vi "AeroQuadUploader.vi"(11 "Com Port":refnum<visa-resource-name>="<Select Com Port>") -> (3 "Com Port Out":refnum<visa-resource-name>)   [LabVIEW 2010]
uses:
  <vilib>/Utility/config.llb/Config Data RefNum.ctl
  <vilib>/Utility/config.llb/Read Key (Double).vi
  <vilib>/Utility/config.llb/Read Key (Boolean).vi
  <vilib>/Utility/config.llb/Read Key (Path).vi
  <vilib>/Utility/config.llb/Read Key (String).vi
  <vilib>/Utility/config.llb/Write Key (Path).vi
  <vilib>/Utility/config.llb/Write Key (Boolean).vi
  <vilib>/Utility/config.llb/NI_LVConfig.lvlib
panel:
  in  "Settings":bool
  in  "Update":bool
  in  "Done":bool
  in  "Upload":bool
  in  "Flight Control Board":u16(ring) items=["AeroQuad v2.1", "AeroQuad v2.0", "AeroQuad Mini", "AeroQuad v1.8 or greater", "AeroQuad v1.0", "AeroQuad v1.0 with IDG gyro", "Wii sensors", "Paris v3", "AeroQuad v1.0 with Arduino Mega", "AeroQuad with Arduino Mega and Wii sensors", "ArduCopter", "AeroQuad with CHR6DM", "APM/OilPan with CHR6DM"]
  in  "Next":bool
  in  "Previous":bool
  in  "FlightConfig":u16(ring) caption="Flight Configuration" items=["Quad X", "Quad +", "Y4", "Tri", "Hexa X", "Hexa +", "Y6", "Octo X", "Octo +", "Octo X8X"]
  out "Description":string
  in  "Options":i32(listbox) caption="Flight Options"
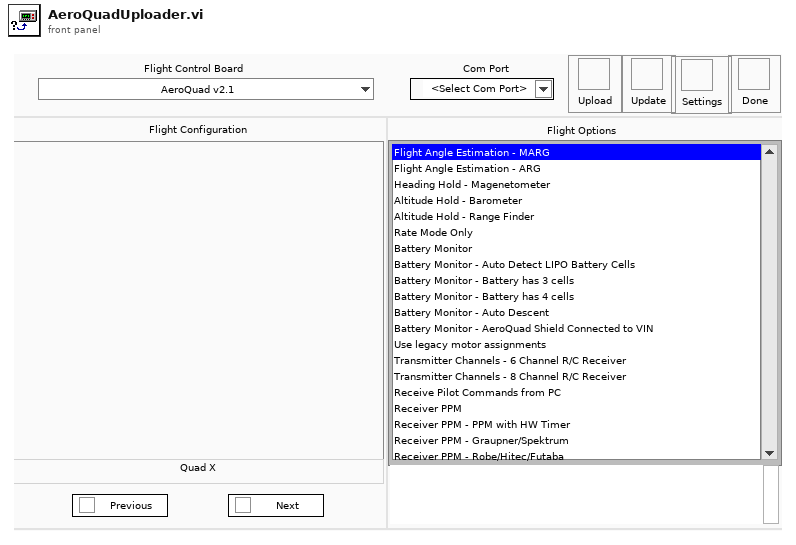
[diagram p1: front panel]
types:
  T1 = typedef "NI_LVConfig.lvlib/Config Data RefNum.ctl" = refnum<k1>
  T2 = cluster{"Error":errorcluster, "ConfigRef":T1, "OptionName":string[], "OptionDesc":string[], "FlightBoard":string[], "ValidOptions":string[][], "ValidBoards":string[], "OptionID":string[], "DefaultOptions":string[][], "DefaultBoards":string[], "FlightSWPath":path, "IDEPath":path, "Debug":bool, "TempPath":path, "Processors":string[][], "ProcessorID":string[], "ConfigID":string[], "ConfigName":string[], "WorkingPath":path, "DebugMsg":bool, "MCU":string, "Mac":bool, "Delay":dbl}
  T3 = enum16{"Left Button", "Center Button", "Right Button", "Window Close"}
  T4 = enum32{"invalid app kind", "Development System", "Run Time System", "Student Edition", "Embedded LabVIEW", "Evaluation", "Custom"}
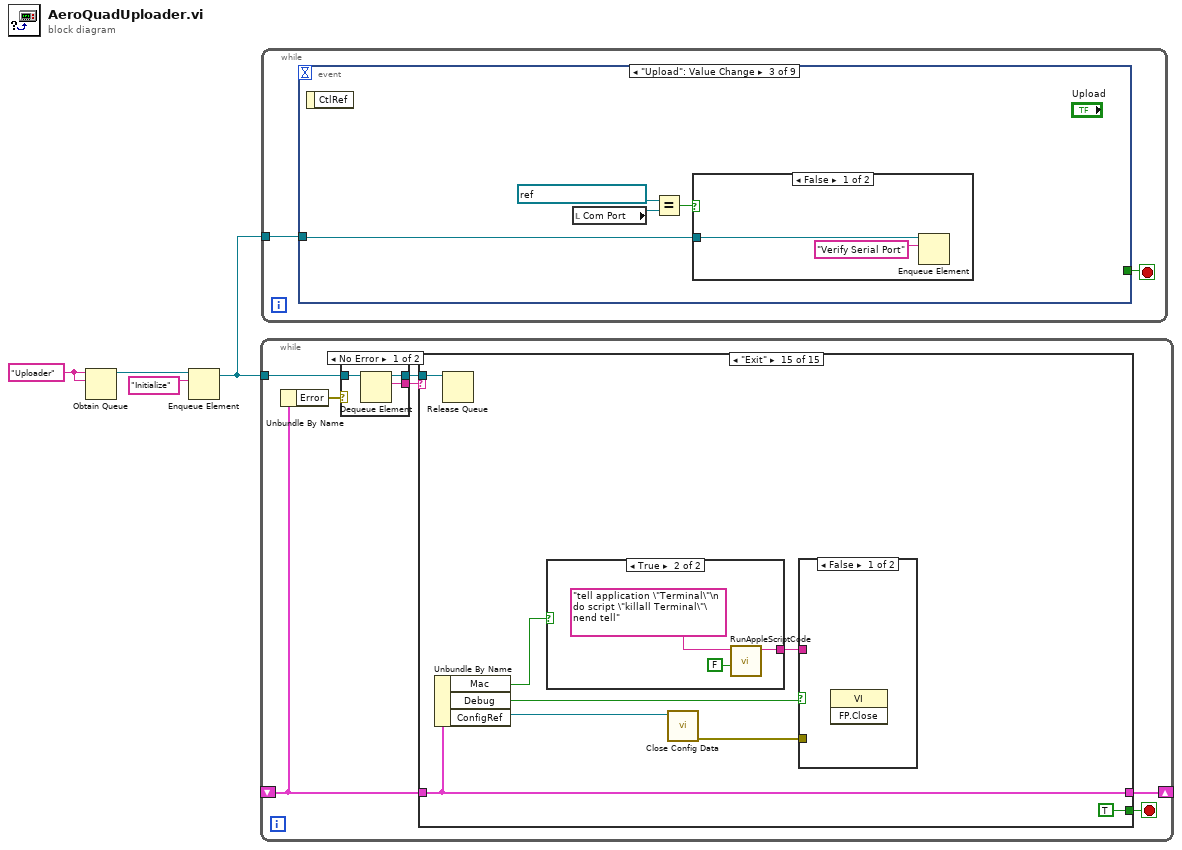
[diagram p0: block diagram]
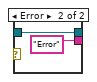
[diagram p2: hidden frame]
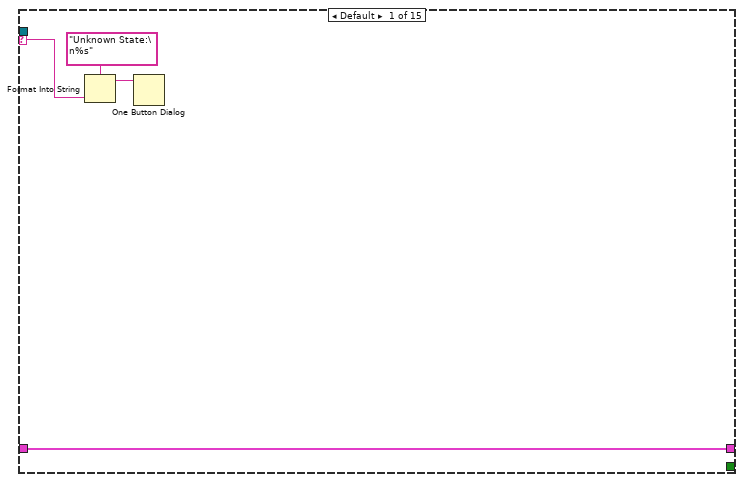
[diagram p3: hidden frame]
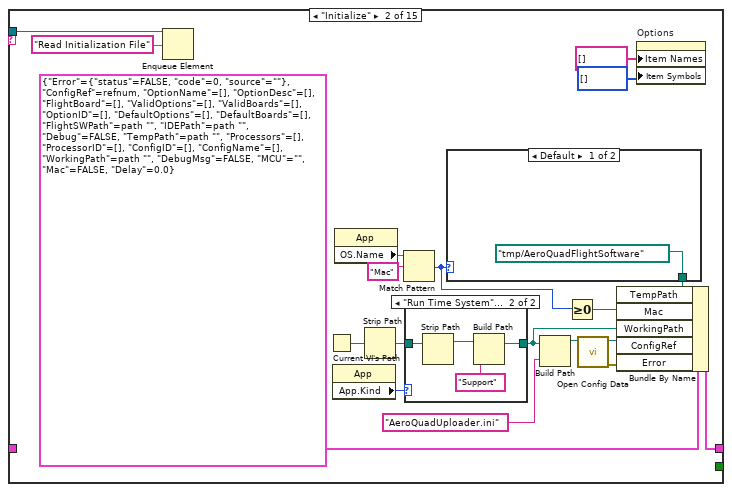
[diagram p4: hidden frame]
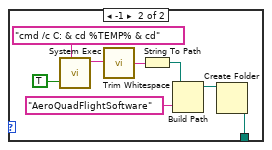
[diagram p5: hidden frame]
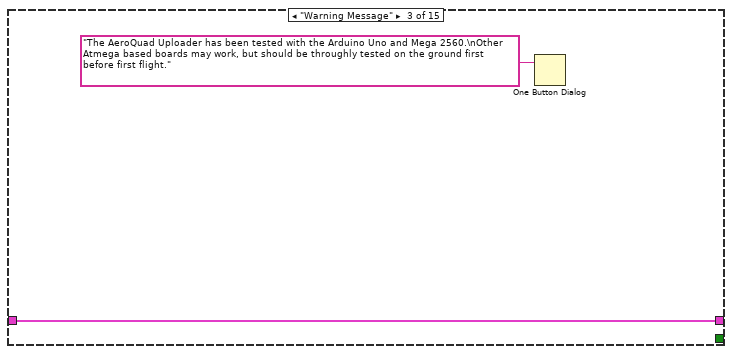
[diagram p7: hidden frame]
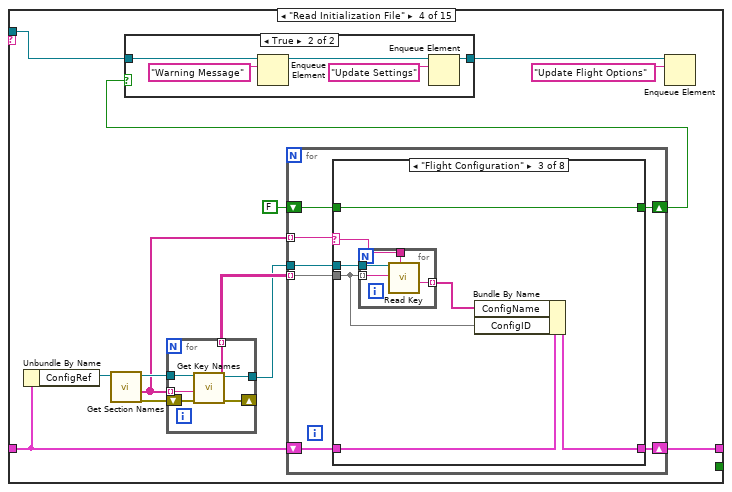
[diagram p8: hidden frame]
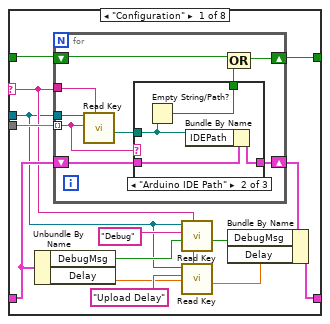
[diagram p10: hidden frame]
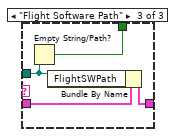
[diagram p12: hidden frame]
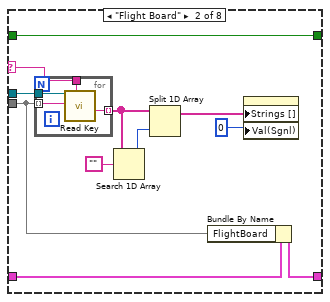
[diagram p13: hidden frame]
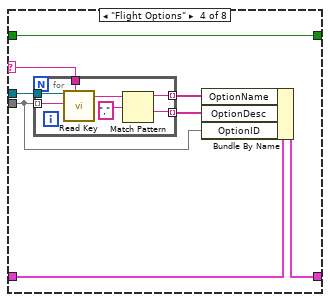
[diagram p14: hidden frame]
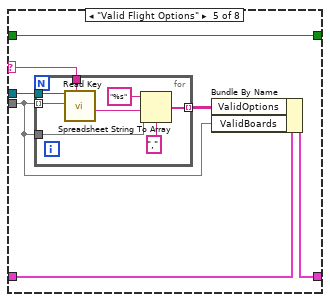
[diagram p15: hidden frame]
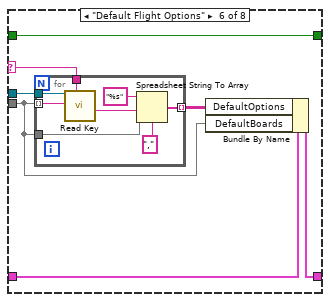
[diagram p16: hidden frame]
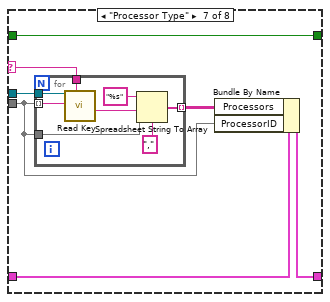
[diagram p17: hidden frame]
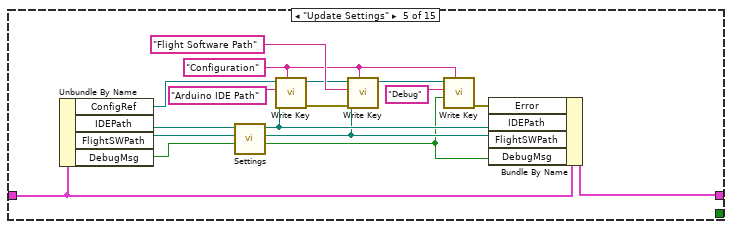
[diagram p19: hidden frame]
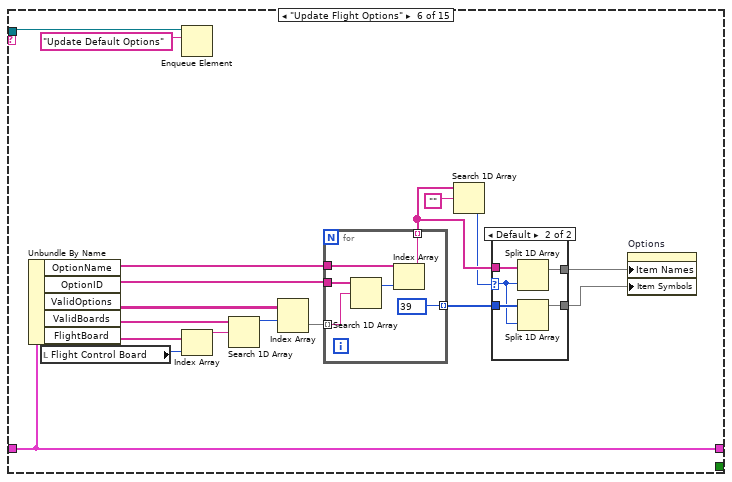
[diagram p20: hidden frame]
diagram:
  w4 = "Uploader" ("name (unnamed)")
  n1 = Obtain Queue(name (unnamed)=w4, element data type=w4) -> (queue out=w3:refnum<queue>)  [unwired: 3 in, 2 out]
  n2 = Enqueue Element(queue=w3, element="Initialize") -> (queue out=w1:refnum<queue>)  [unwired: 2 in, 2 out]
  n3 = while {
    tunnel: w1 -> [w11]
    shift-right: [w8] -> _
    shift-left: _ -> [w7]
    stop <- w9 stop-if-true
    n4 = Unbundle By Name(w7) -> ("Error"=w6:errorcluster)
    n5 = case shown="No Error" w6 {
      tunnel: w11 -> [w14 w15]
      tunnel: [w13 "Error" ("name (unnamed)")] -> w10
      tunnel: [w12 w15] -> w5
      frame No Error {
        n6 = Dequeue Element(queue=w14) -> (queue out=w12:refnum<queue>, element=w13:string)  [unwired: 2 in, 2 out]
      }
      frame Error {
      }
    }
    n7 = case shown="\"Exit\"" w10 {
      tunnel: w5 -> [_ w31 _ w57 _ w226 _ _ w290 w345 w393 w446 _ w586 w597]
      selector: w10 -> [w18 _ _ _ _ _ _ _ _ _ _ _ _ _ _]
      tunnel: [_ _ _ _ _ _ _ _ _ _ _ _ _ _ TRUE] -> w9
      tunnel: [w20 w33 w55 w61 w224 w242 w269 w287 w288 w343 w389 w448 w505 w589 w599] -> w8
      tunnel: w7 -> [w20 _ w55 w62 w223 w242 w269 w287 w288 w340 w390 w449 w506 w590 w599]
      frame Default {
        n8 = Format Into String(format string="Unknown State:\n%s", w18) -> (resulting string=w17:string)  [unwired: 2 in, 1 out]
        n9 = One Button Dialog(message=w17) -> ()  [unwired: 1 in, 1 out]
      }
      frame "Initialize" {
        n10 = Enqueue Element(queue=w31, element="Read Initialization File") -> ()  [unwired: 2 in, 3 out]
        n11 = Current VI's Path() -> (path=w37:path)
        n12 = property class="App"() -> ("App.Kind"=w35:T4)  [unwired: 2 in, 2 out]
        n13 = property class="App"() -> ("OS.Name"=w25:string)  [unwired: 2 in, 2 out]
        n14 = Strip Path(path=w37) -> (stripped path=w36:path)  [unwired: 1 out]
        n15 = Match Pattern(string=w25, regular expression="Mac") -> (offset past match=w22:i32)  [unwired: 1 in, 3 out]
        n16 = case shown="\"Run Time System\", Default" w35 {
          tunnel: w36 -> [w49 w53]
          tunnel: [w49 w52] -> w26
          frame "Development System" {
          }
          frame "Run Time System", Default {
            n17 = Strip Path(path=w53) -> (stripped path=w51:path)  [unwired: 1 out]
            n18 = Build Path(base path=w51, name or relative path="Support") -> (appended path=w52:path)
          }
        }
        n19 = case shown="Default" w22 {
          tunnel: [path "/tmp/AeroQuadFlightSoftware" ("created path") w42] -> w23
          frame Default {
          }
          frame -1 {
            n20 = call <vilib>:"System Exec.vi"("run minimized? (F)"=TRUE, "command line"="cmd /c C: & cd %TEMP% & cd") -> ("standard output"=w44:string)  [unwired: 6 in, 3 out]
            n21 = call <vilib>:"Trim Whitespace.vi"("string"=w44) -> ("trimmed string"=w43:string)  [unwired: 1 in]
            n22 = String To Path(string=w43) -> (path=w46:path)
            n23 = Build Path(base path=w46, name or relative path="AeroQuadFlightSoftware") -> (appended path=w45:path)
            n24 = Create Folder(path (use dialog)=w45) -> (created path=w42:path)  [unwired: 2 in, 2 out]
          }
        }
        n25 = Build Path(base path=w26, name or relative path="AeroQuadUploader.ini") -> (appended path=w39:path)
        n26 = Greater Or Equal To 0?(x=w22) -> (x >= 0?=w21:bool)
        n27 = call <vilib>:"Open Config Data.vi"("configuration file path"=w39) -> ("error out"=w32:errorcluster, "refnum"=w27:T1)  [unwired: 8 in, 1 out]
        n28 = Bundle By Name(cluster=T2 {"Error"={"status"=FALSE, "code"=0, "source"=""}, "ConfigRef"=refnum, "OptionName"=[], "OptionDesc"=[], "FlightBoard"=[], "ValidOptions"=[], "ValidBoards"=[], "OptionID"=[], "DefaultOptions"=[], "DefaultBoards"=[], "FlightSWPath"=path "", "IDEPath"=path "", "Debug"=FALSE, "TempPath"=path "", "Processors"=[], "ProcessorID"=[], "ConfigID"=[], "ConfigName"=[], "WorkingPath"=path "", "DebugMsg"=FALSE, "MCU"="", "Mac"=FALSE, "Delay"=0.0}, "TempPath"=w23, "Mac"=w21, "WorkingPath"=w26, "ConfigRef"=w27, "Error"=w32) -> (w33:T2)
        n29 = property on="Options" class="LstBox (strict)"("Item Names"=string[] [], "Item Symbols"=i32[] []) -> ()  [unwired: 2 in, 2 out]
      }
      frame "Warning Message" {
        n30 = One Button Dialog(message="The AeroQuad Uploader has been tested with the Arduino Uno and Mega 2560.\nOther Atmega based boards may work, but should be throughly tested on the ground first before first flight.") -> ()  [unwired: 1 in, 1 out]
      }
      frame "Read Initialization File" {
        n31 = Unbundle By Name(w62) -> ("ConfigRef"=w64:T1)
        n32 = call <vilib>:"Get Section Names.vi"("refnum"=w64) -> ("error out"=w65:errorcluster, "section names"=w66:string[], "refnum out"=w68:T1)  [unwired: 8 in]
        n33 = for {
          tunnel: w68 -> [w206]
          tunnel: w66 -> [w205] mode=indexing
          shift-right: [w204] -> _
          shift-left: w65 -> [w207]
          tunnel: [w203] -> w63
          tunnel: [w202] -> w67 mode=indexing
          n34 = call <vilib>:"Get Key Names.vi"("section"=w205, "error in (no error)"=w207, "refnum"=w206) -> ("error out"=w204:errorcluster, "key names"=w202:string[], "refnum out"=w203:T1)  [unwired: 5 in, 1 out]
        }
        n35 = for {
          tunnel: w66 -> [w81] mode=indexing
          tunnel: w67 -> [w80] mode=indexing
          tunnel: w63 -> [w79]
          shift-right: [w77] -> w61
          shift-left: w62 -> [w78]
          shift-right: [w75] -> w56
          shift-left: FALSE -> [w76]
          n36 = case shown="\"Flight Configuration\"" w81 {
            selector: w81 -> [w86 w123 w134 w147 w160 w175 w190 _]
            tunnel: w80 -> [w95 w119 w131 w141 w156 w171 w186 _]
            tunnel: w79 -> [w82 w124 w135 w146 w161 w176 w191 _]
            tunnel: w78 -> [w90 w121 w133 w145 w159 w174 w189 w201]
            tunnel: [w92 w120 w132 w144 w158 w173 w188 w201] -> w77
            tunnel: w76 -> [w88 w114 w129 w140 w155 w170 w185 w200]
            tunnel: [w87 w114 w129 w140 w155 w170 w185 w200] -> w75
            frame "Configuration" {
              n37 = Unbundle By Name(w90) -> ("DebugMsg"=w89:bool, "Delay"=w84:dbl)
              n38 = for {
                tunnel: w82 -> [w104]
                tunnel: w86 -> [w103]
                tunnel: w95 -> [w100] mode=indexing
                shift-right: [w101] -> w93
                shift-left: w90 -> [w102]
                shift-right: [w97] -> w87
                shift-left: w88 -> [w98]
                n39 = call-poly <vilib>:"Read Key.vi"("section"=w103, "key"=w100, "refnum"=w104) -> ("value"=w99:path)  [unwired: 5 in, 3 out]
                n40 = case shown="\"Arduino IDE Path\"" w100 {
                  tunnel: w102 -> [w105 w109 w113]
                  tunnel: [w105 w108 w112] -> w101
                  tunnel: w99 -> [_ w107 w111]
                  tunnel: [_ w106 w110] -> w96
                  frame Default {
                  }
                  frame "Arduino IDE Path" {
                    n41 = Empty String/Path?(string/path=w107) -> (empty?=w106:bool)
                    n42 = Bundle By Name(cluster=w109, "IDEPath"=w107) -> (w108:T2)
                  }
                  frame "Flight Software Path" {
                    n43 = Empty String/Path?(string/path=w111) -> (empty?=w110:bool)
                    n44 = Bundle By Name(cluster=w113, "FlightSWPath"=w111) -> (w112:T2)
                  }
                }
                n45 = Compound Arithmetic op=OR(w98, w96) -> (w97:bool)
              }
              n46 = call-poly <vilib>:"Read Key.vi"("section"=w86, "default value"=w89, "key"="Debug", "refnum"=w82) -> ("value"=w91:bool)  [unwired: 4 in, 3 out]
              n47 = call-poly <vilib>:"Read Key.vi"("section"=w86, "default value"=w84, "key"="Upload Delay", "refnum"=w82) -> ("value"=w83:dbl)  [unwired: 4 in, 3 out]
              n48 = Bundle By Name(cluster=w93, "DebugMsg"=w91, "Delay"=w83) -> (w92:T2)
            }
            frame "Flight Board" {
              n49 = for {
                tunnel: w124 -> [w128]
                tunnel: w123 -> [w127]
                tunnel: w119 -> [w126] mode=indexing
                tunnel: [w125] -> w116 mode=indexing
                n50 = call-poly <vilib>:"Read Key.vi"("section"=w127, "key"=w126, "refnum"=w128) -> ("value"=w125:string)  [unwired: 5 in, 3 out]
              }
              n51 = Search 1D Array(1D array=w116, element="") -> (index of element=w117:i32)  [unwired: 1 in]
              n52 = Split 1D Array(array=w116, index=w117) -> (first subarray=w115:string[])  [unwired: 1 out]
              n53 = Bundle By Name(cluster=w121, "FlightBoard"=w119) -> (w120:T2)
              n54 = property on="Flight Control Board" class="Ring (strict)"("Strings []"=w115, "Val(Sgnl)"=u16 0 ("Value (Signaling)")) -> ()  [unwired: 2 in, 2 out]
            }
            frame "Flight Configuration" {
              n55 = for {
                tunnel: w135 -> [w139]
                tunnel: w134 -> [w138]
                tunnel: w131 -> [w137] mode=indexing
                tunnel: [w136] -> w130 mode=indexing
                n56 = call-poly <vilib>:"Read Key.vi"("section"=w138, "key"=w137, "refnum"=w139) -> ("value"=w136:string)  [unwired: 5 in, 3 out]
              }
              n57 = Bundle By Name(cluster=w133, "ConfigName"=w130, "ConfigID"=w131) -> (w132:T2)
            }
            frame "Flight Options" {
              n58 = for {
                tunnel: w146 -> [w154]
                tunnel: w147 -> [w153]
                tunnel: w141 -> [w152] mode=indexing
                tunnel: [w149] -> w143 mode=indexing
                tunnel: [w148] -> w142 mode=indexing
                n59 = call-poly <vilib>:"Read Key.vi"("section"=w153, "key"=w152, "refnum"=w154) -> ("value"=w150:string)  [unwired: 5 in, 3 out]
                n60 = Match Pattern(string=w150, regular expression=",") -> (before substring=w149:string, after substring=w148:string)  [unwired: 1 in, 2 out]
              }
              n61 = Bundle By Name(cluster=w145, "OptionName"=w143, "OptionDesc"=w142, "OptionID"=w141) -> (w144:T2)
            }
            frame "Valid Flight Options" {
              n62 = for {
                tunnel: w161 -> [w169]
                tunnel: w160 -> [w168]
                tunnel: w156 -> [w167] mode=indexing
                tunnel: w156 -> [w165]
                tunnel: [w162] -> w157 mode=indexing
                n63 = call-poly <vilib>:"Read Key.vi"("section"=w168, "key"=w167, "refnum"=w169) -> ("value"=w164:string)  [unwired: 5 in, 3 out]
                n64 = Spreadsheet String To Array(delimiter (Tab)=",", format string="%s", spreadsheet string=w164, array type (2D Dbl)=w165) -> (array=w162:string[])
              }
              n65 = Bundle By Name(cluster=w159, "ValidOptions"=w157, "ValidBoards"=w156) -> (w158:T2)
            }
            frame "Default Flight Options" {
              n66 = for {
                tunnel: w176 -> [w184]
                tunnel: w175 -> [w183]
                tunnel: w171 -> [w182] mode=indexing
                tunnel: w171 -> [w180]
                tunnel: [w177] -> w172 mode=indexing
                n67 = call-poly <vilib>:"Read Key.vi"("section"=w183, "key"=w182, "refnum"=w184) -> ("value"=w179:string)  [unwired: 5 in, 3 out]
                n68 = Spreadsheet String To Array(delimiter (Tab)=",", format string="%s", spreadsheet string=w179, array type (2D Dbl)=w180) -> (array=w177:string[])
              }
              n69 = Bundle By Name(cluster=w174, "DefaultOptions"=w172, "DefaultBoards"=w171) -> (w173:T2)
            }
            frame "Processor Type" {
              n70 = for {
                tunnel: w191 -> [w199]
                tunnel: w190 -> [w198]
                tunnel: w186 -> [w197] mode=indexing
                tunnel: w186 -> [w195]
                tunnel: [w192] -> w187 mode=indexing
                n71 = call-poly <vilib>:"Read Key.vi"("section"=w198, "key"=w197, "refnum"=w199) -> ("value"=w194:string)  [unwired: 5 in, 3 out]
                n72 = Spreadsheet String To Array(delimiter (Tab)=",", format string="%s", spreadsheet string=w194, array type (2D Dbl)=w195) -> (array=w192:string[])
              }
              n73 = Bundle By Name(cluster=w189, "Processors"=w187, "ProcessorID"=w186) -> (w188:T2)
            }
            frame Default {
            }
          }
        }
        n74 = case shown="True" w56 {
          tunnel: [w69 w74] -> w58
          tunnel: w57 -> [w69 w71]
          frame False {
          }
          frame True {
            n75 = Enqueue Element(queue=w71, element="Warning Message") -> (queue out=w70:refnum<queue>)  [unwired: 2 in, 2 out]
            n76 = Enqueue Element(queue=w70, element="Update Settings") -> (queue out=w74:refnum<queue>)  [unwired: 2 in, 2 out]
          }
        }
        n77 = Enqueue Element(queue=w58, element="Update Flight Options") -> ()  [unwired: 2 in, 3 out]
      }
      frame "Update Settings" {
        w211 = "Configuration" ("section")
        n78 = Unbundle By Name(w223) -> ("ConfigRef"=w222:T1, "IDEPath"=w215:path, "FlightSWPath"=w214:path, "DebugMsg"=w213:bool)
        n79 = call "Settings.vi"("Debug"=w213, "AeroQuad Flight Software Folder"=w214, "Location of Arduino Application"=w215) -> ("Debug Out"=w208:bool, "Flight Software Path"=w216:path, "IDE Path"=w217:path)  [unwired: 6 in]
        n80 = call-poly <vilib>:"Write Key.vi"("section"=w211, "value"=w217, "key"="Arduino IDE Path", "refnum"=w222) -> ("error out"=w221:errorcluster, "refnum out"=w218:T1)  [unwired: 5 in, 1 out]
        n81 = call-poly <vilib>:"Write Key.vi"("section"=w211, "error in (no error)"=w221, "value"=w216, "key"="Flight Software Path", "refnum"=w218) -> ("refnum out"=w210:T1)  [unwired: 4 in, 2 out]
        n82 = call-poly <vilib>:"Write Key.vi"("section"=w211, "value"=w208, "key"="Debug", "refnum"=w210) -> ("error out"=w212:errorcluster)  [unwired: 5 in, 2 out]
        n83 = Bundle By Name(cluster=w223, "Error"=w212, "IDEPath"=w217, "FlightSWPath"=w216, "DebugMsg"=w208) -> (w224:T2)
      }
      frame "Update Flight Options" {
        n84 = Unbundle By Name(w242) -> ("OptionName"=w233:string[], "OptionID"=w234:string[], "ValidOptions"=w237:string[][], "ValidBoards"=w238:string[], "FlightBoard"=w240:string[])
        n85 = local read "Flight Control Board"() -> (w241:u16)
        n86 = Enqueue Element(queue=w226, element="Update Default Options") -> ()  [unwired: 2 in, 3 out]
        n87 = Index Array(array=w240, index=w241) -> (element=w239:string)
        n88 = Search 1D Array(1D array=w238, element=w239) -> (index of element=w236:i32)  [unwired: 1 in]
        n89 = Index Array(array=w237, index (row)=w236) -> (element=w235:string[])  [unwired: 1 in]
        n90 = for {
          tunnel: w235 -> [w254] mode=indexing
          tunnel: w234 -> [w255]
          tunnel: w233 -> [w253]
          tunnel: [w251] -> w231 mode=indexing
          tunnel: [39] -> w230 mode=indexing
          n91 = Search 1D Array(1D array=w255, element=w254) -> (index of element=w252:i32)  [unwired: 1 in]
          n92 = Index Array(array=w253, index=w252) -> (element=w251:string)
        }
        n93 = Search 1D Array(1D array=w231, element="") -> (index of element=w227:i32)  [unwired: 1 in]
        n94 = case shown="Default" w227 {
          selector: w227 -> [_ w245]
          tunnel: w231 -> [w244 w249]
          tunnel: w230 -> [w243 w248]
          tunnel: [w244 w247] -> w229
          tunnel: [w243 w246] -> w228
          frame -1 {
          }
          frame Default {
            n95 = Split 1D Array(array=w249, index=w245) -> (first subarray=w247:string[])  [unwired: 1 out]
            n96 = Split 1D Array(array=w248, index=w245) -> (first subarray=w246:i32[])  [unwired: 1 out]
          }
        }
        n97 = property on="Options" class="LstBox (strict)"("Item Names"=w229, "Item Symbols"=w228) -> ()  [unwired: 2 in, 2 out]
      }
      frame "Update Default Options" {
        w256 = 0 ("Value (Signaling)")
        n98 = Unbundle By Name(w269) -> ("OptionName"=w260:string[], "OptionID"=w262:string[], "DefaultOptions"=w264:string[][], "DefaultBoards"=w265:string[], "FlightBoard"=w268:string[])
        n99 = local read "Flight Control Board"() -> (w267:u16)
        n100 = Index Array(array=w268, index=w267) -> (element=w266:string)
        n101 = property on="Options" class="LstBox (strict)"() -> ("Item Symbols"=w259:i32[], "Item Names"=w258:string[])  [unwired: 2 in, 2 out]
        n102 = Search 1D Array(1D array=w265, element=w266) -> (index of element=w263:i32)  [unwired: 1 in]
        n103 = Index Array(array=w264, index (row)=w263) -> (element=w261:string[])  [unwired: 1 in]
        n104 = for {
          tunnel: w262 -> [w279]
          tunnel: w261 -> [w278] mode=indexing
          tunnel: w260 -> [w277]
          tunnel: w258 -> [w272]
          shift-right: [w270] -> w257
          shift-left: w259 -> [w273]
          n105 = Search 1D Array(1D array=w279, element=w278) -> (index of element=w276:i32)  [unwired: 1 in]
          n106 = Index Array(array=w277, index=w276) -> (element=w271:string)
          n107 = Search 1D Array(1D array=w272, element=w271) -> (index of element=w274:i32)  [unwired: 1 in]
          n108 = Replace Array Subset(array=w273, new element=40, index=w274) -> (w270:i32[])
        }
        n109 = property on="Options" class="LstBox (strict)"("Item Symbols"=w257, "Val(Sgnl)"=w256, "Top Row"=w256) -> ()  [unwired: 2 in, 2 out]
      }
      frame "Update Flight Option Description" {
        n110 = Unbundle By Name(w287) -> ("OptionDesc"=w282:string[], "OptionName"=w284:string[])
        n111 = property on="Options" class="LstBox (strict)"() -> ("Item Names"=w285:string[], "Value"=w286:i32)  [unwired: 2 in, 2 out]
        n112 = Index Array(array=w285, index=w286) -> (element=w283:string)
        n113 = Search 1D Array(1D array=w284, element=w283) -> (index of element=w281:i32)  [unwired: 1 in]
        n114 = Index Array(array=w282, index=w281) -> (element=→"Description":string)
      }
      frame "Verify Serial Port" {
        n115 = while {
          tunnel: [w293] -> w289
          i -> [w294]
          stop <- w295 stop-if-true
          n116 = case shown="0" w294 {
            tunnel: [TRUE ("T button?") w301] -> w296
            frame Default {
            }
            frame 0 {
              n117 = Two Button Dialog(message="Verify correct serial port is selected.  Flight board lights should blink quickly when the \"Test\" button is selected.\n\nDo you want to test or proceed with the upload?", 1:"Upload" ("F button name (\"Cancel\")"), 2:"Test" ("T button name (\"OK\")")) -> (T button?=w301:bool)
            }
          }
          n118 = case shown="True" w296 {
            selector: w296 -> [w302 _]
            tunnel: [w303 w306] -> w295
            tunnel: [w302 w305] -> w293
            frame False {
              n119 = Not(x=w302) -> (.not. x?=w303:bool)
            }
            frame True {
              n120 = local read "Com Port"() -> (w304:refnum<visa-resource-name>)
              n121 = call "TestUsbSerialPort.vi"("Serial Port To Test"=w304) -> ("Error Out"=w307:errorcluster)  [unwired: 9 in, 1 out]
              n122 = case shown="No Error" w307 {
                tunnel: [w312 w317] -> w306
                tunnel: [w309 w317] -> w305
                frame No Error {
                  n123 = call <vilib>:"Three Button Dialog.vi"("Justify Message (Left)"=enum16{"Left", "Center", "Right"}."Center", "Right Button Text (\"Cancel\")"="Choose Different Port" ("F button name (\"Cancel\")"), "Center Button Text (\"No\")"="Test Again" ("T button name (\"OK\")"), "message"="Did lights blink quickly?") -> ("Which Button?"=w308:T3)  [unwired: 7 in]
                  n124 = Equal?(x=w308, y=T3."Right Button" ("Which Button?")) -> (x = y?=w309:bool)
                  n125 = Not Equal?(x=T3."Center Button" ("Which Button?"), y=w308) -> (x != y?=w312:bool)
                }
                frame Error {
                  w317 = TRUE ("T button?")
                  n126 = One Button Dialog(message="Communication error detected.  Choose another serial port.") -> ()  [unwired: 1 in, 1 out]
                }
              }
            }
          }
        }
        n127 = case shown="False" w289 {
          tunnel: w290 -> [w292 _]
          frame False {
            n128 = Enqueue Element(queue=w292, element="Copy Flight Software to Temp Folder") -> ()  [unwired: 2 in, 3 out]
          }
          frame True {
          }
        }
      }
      frame "Copy Flight Software to Temp Folder" {
        # "Copy Makefile"
        # "Clear Temp Folder"
        n129 = Unbundle By Name(w340) -> ("Mac"=w325:bool, "TempPath"=w335:path, "Error"=w334:errorcluster, "FlightSWPath"=w323:path, "WorkingPath"=w333:path)
        n130 = call <vilib>:"Set Busy.vi"("error in (no error)"=w334) -> ("error out"=w336:errorcluster)  [unwired: 9 in, 1 out]
        n131 = Enqueue Element(queue=w345, element="Generate Makefile") -> ()  [unwired: 2 in, 3 out]
        n132 = Delete(path (use dialog)=w335, entire hierarchy (F)=TRUE, error in=w336) -> (deleted path=w324:path, error out=w320:errorcluster)  [unwired: 2 in, 1 out]
        n133 = Build Path(base path=w333, name or relative path="Makefile") -> (appended path=w337:path)
        n134 = case shown="True" w325 {
          tunnel: [w350 w356] -> w322
          tunnel: [path "C:/" ("working directory") path "\\" ("working directory")] -> w326
          tunnel: w324 -> [w347 w357]
          tunnel: w323 -> [w349 w358]
          tunnel: [w346 path "/tmp/AeroQuadFlightSoftware/ready" ("appended path")] -> w321
          tunnel: w320 -> [_ _]
          frame False {
            n135 = Format Into String(format string="cmd /c xcopy \"%s\" \"%s\" /I /E /Y & echo 1 > %s\\\\ready", w349, w347, w347) -> (resulting string=w350:string)  [unwired: 2 in, 1 out]
            n136 = Build Path(base path=w347, name or relative path="ready") -> (appended path=w346:path)
          }
          frame True {
            n137 = call "Mac2LinuxPath.vi"("Mac Path"=w358) -> ("Linux Path"=w354:string)  [unwired: 9 in, 1 out]
            n138 = call "Mac2LinuxPath.vi"("Mac Path"=w357) -> ("Linux Path"=w355:string)  [unwired: 9 in, 1 out]
            n139 = Format Into String(format string="mkdir %s; cp -R %s/* %s; touch %s/ready", w355, w354, w355, w355) -> (resulting string=w356:string)  [unwired: 2 in, 1 out]
          }
        }
        n140 = call <vilib>:"System Exec.vi"("run minimized? (F)"=TRUE, "wait until completion? (T)"=FALSE, "working directory"=w326, "command line"=w322) -> ("error out"=w329:errorcluster)  [unwired: 4 in, 3 out]
        n141 = Build Path(base path=w324, name or relative path="AeroQuad") -> (appended path=w332:path)
        n142 = while {
          tunnel: w321 -> [w370]
          tunnel: w329 -> [w369]
          tunnel: [w367] -> w328
          i -> [w365]
          stop <- w362 stop-if-true
          n143 = call <vilib>:"Check if File or Folder Exists.vi"("error in (no error)"=w369, "path"=w370) -> ("error out"=w367:errorcluster, "file or folder exists?"=w368:bool)  [unwired: 7 in, 1 out]
          n144 = Unbundle By Name(w367) -> ("status"=w366:bool)
          n145 = Greater?(x=w365, y=150) -> (0:w363:bool)
          n146 = Compound Arithmetic op=OR(w368, w366, w363) -> (w362:bool)
          n147 = Wait Until Next ms Multiple(millisecond multiple=u32 1000) -> ()  [unwired: 1 out]
        }
        n148 = Copy(8:w328, 9:TRUE ("overwrite (F)"), 10:w332, 11:w337) -> (0:w319:errorcluster)  [unwired: 1 in, 2 out]
        n149 = Bundle By Name(cluster=w340, "Error"=w319) -> (w343:T2)
        n150 = call <vilib>:"Clear Errors.vi"("error in (no error)"=w319) -> ("error out"=w338:errorcluster)  [unwired: 6 in]
        n151 = call <vilib>:"Unset Busy.vi"("error in (no error)"=w338) -> ()  [unwired: 10 in, 1 out]
      }
      frame "Generate Makefile" {
        n152 = Unbundle By Name(w390) -> ("Mac"=w374:bool, "IDEPath"=w384:path, "TempPath"=w380:path, "ProcessorID"=w400:string[], "Processors"=w399:string[][], "FlightBoard"=w397:string[])
        n153 = Unbundle By Name(w390) -> ("TempPath"=w392:path)
        n154 = Select(t="/bin\nPORT = /dev/tty.usb*", s=w374, f="$(INSTALL_DIR)/hardware/tools/avr/utils/bin") -> (s? t:f=w371:string)
        n155 = Index Array(array=w397, index="Flight Control Board") -> (element=w382:string)
        n156 = for {
          tunnel: w400 -> [w428] mode=indexing
          tunnel: w399 -> [w429] mode=indexing
          tunnel: w382 -> [w430]
          tunnel: [w428] -> w383
          stop <- w427 continue-if-true
          n157 = Search 1D Array(1D array=w429, element=w430) -> (index of element=w426:i32)  [unwired: 1 in]
          n158 = Less Than 0?(x=w426) -> (x < 0?=w427:bool)
        }
        n159 = Build Path(base path=w392, name or relative path="AeroQuad") -> (appended path=w378:path)
        n160 = case shown="Default" w382 {
          tunnel: [57600 115200] -> w381
          frame "AeroQuad_Mini" {
          }
          frame Default {
          }
        }
        n161 = case shown="True" w374 {
          tunnel: w384 -> [w413 w414]
          tunnel: w380 -> [w410 w419]
          tunnel: [w402 w418] -> w376
          tunnel: [w405 w417] -> w375
          frame False {
            w407 = "/" ("replace string (\"\")")
            w408 = "\\" ("search string")
            n162 = call "GetShortPathName.vi"("Long Path In:"=w413) -> ("Short Path Out:"=w412:path)  [unwired: 8 in, 2 out]
            n163 = call "GetShortPathName.vi"("Long Path In:"=w410) -> ("Short Path Out:"=w411:path)  [unwired: 8 in, 2 out]
            n164 = Path To String(path=w412) -> (string=w404:string)
            n165 = Path To String(path=w411) -> (string=w403:string)
            n166 = Search and Replace String(replace all?=TRUE ("replace all? (F)"), input string=w404, search string=w408, replace string=w407) -> (result string=w402:string)  [unwired: 4 in, 3 out]
            n167 = Search and Replace String(replace all?=TRUE ("replace all? (F)"), input string=w403, search string=w408, replace string=w407) -> (result string=w405:string)  [unwired: 4 in, 3 out]
          }
          frame True {
            n168 = Build Path(base path=w414, name or relative path=":Arduino.app:Contents:Resources:Java") -> (appended path=w416:path)
            n169 = call "Mac2LinuxPath.vi"("Mac Path"=w416) -> ("Linux Path"=w418:string)  [unwired: 9 in, 1 out]
            n170 = call "Mac2LinuxPath.vi"("Mac Path"=w419) -> ("Linux Path"=w417:string)  [unwired: 9 in, 1 out]
          }
        }
        n171 = Build Path(base path=w378, name or relative path="config.mk") -> (appended path=w377:path)
        n172 = local read "Com Port"() -> (w385:refnum<visa-resource-name>)
        n173 = case "Put this into INI file\nwhen read for Maple" shown="\"atmega2560\", Default" w383 {
          tunnel: ["$(INSTALL_DIR)/hardware/arduino/variants/standard" "$(INSTALL_DIR)/hardware/arduino/variants/mega"] -> w396
          tunnel: ["arduino" "stk500v2"] -> w395
          frame "atmega328p" {
          }
          frame "atmega2560", Default {
          }
        }
        n174 = call "ListLibraryFolders.vi"("Mac"=w374, "Path"=w380) -> ("Include List"=w387:string)  [unwired: 8 in, 1 out]
        n175 = Format Into String(format string="INSTALL_DIR = %s\nAQ = %s\nAQ_INCS = %s\nPORT = %s\nUPLOAD_RATE = %d\nMCU = %s\nVARIANTS = %s\nAVRDUDE_PROGRAMMER = %s\nAVR_UTILS_PATH = %s\n", w376, w375, w387, w385, w381, w383, w396, w395, w371) -> (resulting string=w391:string)  [unwired: 2 in, 1 out]
        n176 = call "AutoRenameFile.vi"("Contents"=w391, "Filename"=w377) -> ("error out"=w388:errorcluster)  [unwired: 9 in]
        n177 = Bundle By Name(cluster=w390, "Error"=w388, "MCU"=w383) -> (w389:T2)
        n178 = Enqueue Element(queue=w393, element="Generate UserConfiguration.h") -> ()  [unwired: 2 in, 3 out]
      }
      frame "Generate UserConfiguration.h" {
        w440 = "#define %s\n" ("format string")
        n179 = property on="FlightConfig" class="Ring (strict)"() -> ("Strings []"=w456:string[], "Value"=w457:u16)  [unwired: 2 in, 2 out]
        n180 = Unbundle By Name(w449) -> ("ConfigName"=w444:string[], "ConfigID"=w443:string[], "FlightBoard"=w438:string[], "OptionID"=w460:string[], "OptionName"=w461:string[], "TempPath"=w434:path)
        n181 = Index Array(array=w456, index=w457) -> (element=w455:string)
        n182 = Search 1D Array(1D array=w444, element=w455) -> (index of element=w454:i32)  [unwired: 1 in]
        n183 = Enqueue Element(queue=w446, element="Upload Flight Software") -> ()  [unwired: 2 in, 3 out]
        n184 = property on="Options" class="LstBox (strict)"() -> ("Item Names"=w462:string[], "Item Symbols"=w459:i32[])  [unwired: 2 in, 2 out]
        n185 = Index Array(array=w443, index=w454) -> (element=w453:string)
        n186 = Build Path(base path=w434, name or relative path="AeroQuad") -> (appended path=w435:path)
        n187 = local read "Flight Control Board"() -> (w442:u16)
        n188 = Index Array(array=w438, index=w442) -> (element=w441:string)
        n189 = Format Into String(format string=w440, initial string="/*\n    UserConfiguration.h\n    This file is auto-generated by the AeroQuad Uploader\n    This defines all the user configurable items for the AeroQuad Software\n*/\n\r#ifndef _USER_CONFIG_H_\n#define _USER_CONFIG_H_\r\n\n", w441) -> (resulting string=w439:string)  [unwired: 1 in, 1 out]
        n190 = Format Into String(format string=w440, initial string=w439, w453) -> (resulting string=w437:string)  [unwired: 1 in, 1 out]
        n191 = for {
          tunnel: w462 -> [w469]
          tunnel: w461 -> [w468]
          tunnel: w460 -> [w467]
          tunnel: w459 -> [w466] mode=indexing
          shift-right: [w463] -> w458
          shift-left: w437 -> [w464]
          i -> [w465]
          n192 = case shown="40" w466 {
            tunnel: w469 -> [_ w482]
            tunnel: w468 -> [_ w481]
            tunnel: w467 -> [_ w479]
            tunnel: w465 -> [_ w477]
            tunnel: w464 -> [w470 w476]
            tunnel: [w470 w473] -> w463
            frame Default {
            }
            frame 40 {
              n193 = Index Array(array=w482, index=w477) -> (element=w480:string)
              n194 = Search 1D Array(1D array=w481, element=w480) -> (index of element=w478:i32)  [unwired: 1 in]
              n195 = Index Array(array=w479, index=w478) -> (element=w474:string)
              n196 = Format Into String(format string="#define %s", initial string=w476, w474) -> (resulting string=w472:string)  [unwired: 1 in, 1 out]
              n197 = Concatenate Strings(w472, "\r\n") -> (w473:string)
            }
          }
        }
        n198 = Build Path(base path=w435, name or relative path="UserConfiguration.h") -> (appended path=w451:path)
        n199 = Concatenate Strings(w458, "\r\n", "#endif" ("string")) -> (w450:string)
        n200 = call "AutoRenameFile.vi"("Contents"=w450, "Filename"=w451) -> ("error out"=w452:errorcluster)  [unwired: 9 in]
        n201 = Bundle By Name(cluster=w449, "Error"=w452) -> (w448:T2)
      }
      frame "Upload Flight Software" {
        n202 = Unbundle By Name(w506) -> ("Mac"=w497:bool, "IDEPath"=w498:path, "TempPath"=w509:path, "MCU"=w504:string, "DebugMsg"=w503:bool, "Delay"=w491:dbl)
        n203 = property on="Flight Control Board" class="Ring (strict)"() -> ("Strings []"=w500:string[], "Value"=w501:u16)  [unwired: 2 in, 2 out]
        n204 = Index Array(array=w500, index=w501) -> (element=w499:string)
        n205 = call "GetShortPathName.vi"("Long Path In:"=w498) -> ("Short Path Out:"=w496:path)  [unwired: 8 in, 2 out]
        n206 = case shown="True" w497 {
          tunnel: [w513 w521] -> w487
          tunnel: w496 -> [w518 w522]
          tunnel: [w515 w523] -> w495
          tunnel: [TRUE ("wait until completion? (T)") FALSE ("wait until completion? (T)")] -> w486
          frame True {
            n207 = call "Mac2LinuxPath.vi"("Mac Path"=w518) -> ("Linux Path"=w510:string)  [unwired: 9 in, 1 out]
            n208 = Format Into String(format string="tell application \"Terminal\"\n  activate\n  do script \"cd /tmp/AeroQuadFlightSoftware/AeroQuad; %s/Arduino.app/Contents/Resources/Java/hardware/tools/avr/bin/make clean ; %s/Arduino.app/Contents/Resources/Java/hardware/tools/avr/bin/make ; touch upload; exit\"\nend tell", w510, w510) -> (resulting string=w516:string)  [unwired: 2 in, 1 out]
            n209 = call "RunAppleScriptCode.vi"("Input String"=w516) -> ("Results"=w515:string)  [unwired: 8 in, 2 out]
            n210 = Format Into String(format string="tell application \"Terminal\"\n  do script \"cd /tmp/AeroQuadFlightSoftware/AeroQuad; %s/Arduino.app/Contents/Resources/Java/hardware/tools/avr/bin/make sizeafter upload; read; killall Terminal\"\nend tell", w510) -> (resulting string=w514:string)  [unwired: 2 in, 1 out]
            n211 = call "RunAppleScriptCode.vi"("Input String"=w514) -> ("Results"=w513:string)  [unwired: 8 in, 2 out]
          }
          frame False {
            n212 = Format Into String(format string="cmd /c @echo Starting flight software compile... & PATH=%s\\\\hardware\\\\tools\\\\avr\\\\utils\\\\bin;%%PATH%% & cmd /c make clean & cmd /c make & echo 1 > upload", w522) -> (resulting string=w523:string)  [unwired: 2 in, 1 out]
            n213 = Format Into String(format string="cmd /c @echo Uploading flight software to microcontroller... & @ PATH=%s\\\\hardware\\\\tools\\\\avr\\\\utils\\\\bin;%%PATH%% & cmd /c make sizeafter upload & pause", w522) -> (resulting string=w521:string)  [unwired: 2 in, 1 out]
          }
        }
        n214 = Build Path(base path=w509, name or relative path="AeroQuad") -> (appended path=w488:path)
        n215 = call <vilib>:"Set Busy.vi"() -> ("error out"=w507:errorcluster)  [unwired: 10 in, 1 out]
        n216 = Not(x=w503) -> (.not. x?=w502:bool)
        n217 = call <vilib>:"System Exec.vi"("run minimized? (F)"=w502, "wait until completion? (T)"=w486, "error in (no error)"=w507, "working directory"=w488, "command line"=w495) -> ("error out"=w490:errorcluster)  [unwired: 3 in, 3 out]
        n218 = Build Path(base path=w488, name or relative path="upload") -> (appended path=w493:path)
        n219 = while {
          tunnel: [w579] -> w489
          tunnel: w490 -> [w580]
          tunnel: w493 -> [w576]
          i -> [w582]
          stop <- w583 stop-if-true
          n220 = call <vilib>:"Check if File or Folder Exists.vi"("error in (no error)"=w580, "path"=w576) -> ("error out"=w579:errorcluster, "file or folder exists?"=w584:bool)  [unwired: 7 in, 1 out]
          n221 = Unbundle By Name(w579) -> ("status"=w578:bool)
          n222 = Greater?(x=w582, y=150) -> (0:w577:bool)
          n223 = Compound Arithmetic op=OR(w577, w584, w578) -> (w583:bool)
          n224 = Wait Until Next ms Multiple(millisecond multiple=u32 1000) -> ()  [unwired: 1 out]
        }
        n225 = case "Put this into INI file\nwhen read for Maple" shown="\"atmega328p\"" w504 {
          tunnel: w489 -> [w528 w559]
          tunnel: [w532 w563] -> w485
          tunnel: w499 -> [w526 _]
          tunnel: w491 -> [w525 w556]
          tunnel: w488 -> [w529 w560]
          tunnel: w487 -> [w530 w561]
          tunnel: w486 -> [w531 w557]
          tunnel: [w533 w562] -> w484
          tunnel: "Com Port" -> [w527 w558]
          frame "atmega328p" {
            n226 = case shown="\"AeroQuad Mini\"" w526 {
              tunnel: [w534 w543] -> w533
              tunnel: [w535 w542] -> w532
              tunnel: w531 -> [_ w541]
              tunnel: w530 -> [_ w540]
              tunnel: w529 -> [_ w539]
              tunnel: w528 -> [w535 w538]
              tunnel: w527 -> [w534 w537]
              tunnel: w525 -> [_ w536]
              frame Default {
              }
              frame "AeroQuad Mini" {
                n227 = while {
                  tunnel: [w549] -> w542
                  tunnel: [w547] -> w543
                  tunnel: w538 -> [w555]
                  tunnel: w540 -> [w554]
                  tunnel: w539 -> [w553]
                  tunnel: w537 -> [w552]
                  tunnel: w541 -> [w551]
                  shift-right: [w545] -> _
                  shift-left: w536 -> [w544]
                  stop <- w546 continue-if-true
                  n228 = call "Upload.vi"("wait until completion? (T)"=w551, "Delay Time (s)"=w544, "DTR Delay"=1.0, "error in"=w555, "Serial Port To Test"=w552, "working directory"=w553, "command line"=w554) -> ("error out"=w548:errorcluster, "Serial Port To Test Out"=w547:refnum<visa-resource-name>)  [unwired: 3 in]
                  n229 = call "VerifyUploadDialog.vi"("Delay"=w544, "error in (no error)"=w548) -> ("Delay"=w545:dbl, "Retry"=w546:bool, "error out"=w549:errorcluster)  [unwired: 15 in]
                }
              }
            }
          }
          frame "atmega2560", Default {
            n230 = while {
              tunnel: [w569] -> w563
              tunnel: [w567] -> w562
              tunnel: w559 -> [w575]
              tunnel: w561 -> [w574]
              tunnel: w560 -> [w573]
              tunnel: w558 -> [w572]
              tunnel: w557 -> [w571]
              shift-right: [w565] -> _
              shift-left: w556 -> [w564]
              stop <- w566 continue-if-true
              n231 = call "Upload.vi"("wait until completion? (T)"=w571, "Delay Time (s)"=w564, "DTR Delay"=1.0, "error in"=w575, "Serial Port To Test"=w572, "working directory"=w573, "command line"=w574) -> ("error out"=w568:errorcluster, "Serial Port To Test Out"=w567:refnum<visa-resource-name>)  [unwired: 3 in]
              n232 = call "VerifyUploadDialog.vi"("Delay"=w564, "error in (no error)"=w568) -> ("Delay"=w565:dbl, "Retry"=w566:bool, "error out"=w569:errorcluster)  [unwired: 15 in]
            }
          }
        }
        "Com Port Out" <- w484
        n233 = call <vilib>:"Clear Errors.vi"("error in (no error)"=w485) -> ("error out"=w492:errorcluster)  [unwired: 6 in]
        n234 = Bundle By Name(cluster=w506, "Error"=w492) -> (w505:T2)
        n235 = call <vilib>:"Unset Busy.vi"("error in (no error)"=w492) -> ()  [unwired: 10 in, 1 out]
      }
      frame "Error" {
        n236 = Flush Queue(queue=w586) -> ()  [unwired: 1 in, 3 out]
        n237 = Unbundle By Name(w590) -> ("Error"=w592:errorcluster)
        n238 = call <vilib>:"Simple Error Handler.vi"("error in (no error)"=w592) -> ("error out"=w591:errorcluster)  [unwired: 4 in, 4 out]
        n239 = call <vilib>:"Clear Errors.vi"("error in (no error)"=w591) -> ("error out"=w588:errorcluster)  [unwired: 6 in]
        n240 = call <vilib>:"Unset Busy.vi"("error in (no error)"=w588) -> ("error out"=w587:errorcluster)  [unwired: 10 in]
        n241 = Bundle By Name(cluster=w590, "Error"=w587) -> (w589:T2)
      }
      frame "Exit" {
        n242 = Unbundle By Name(w599) -> ("Mac"=w594:bool, "Debug"=w595:bool, "ConfigRef"=w598:T1)
        n243 = Release Queue(queue=w597) -> ()  [unwired: 2 in, 3 out]
        n244 = case shown="True" w594 {
          tunnel: [_ w602] -> w593
          frame False {
          }
          frame True {
            n245 = call "RunAppleScriptCode.vi"("Run Later"=FALSE, "Input String"="tell application \"Terminal\"\n  do script \"killall Terminal\"\nend tell") -> ("Results"=w602:string)  [unwired: 7 in, 2 out]
          }
        }
        n246 = call <vilib>:"Close Config Data.vi"("refnum"=w598) -> ("error out"=w596:errorcluster)  [unwired: 9 in, 1 out]
        n247 = case shown="False" w595 {
          tunnel: w596 -> [_ _]
          tunnel: w593 -> [_ _]
          frame False {
            n248 = invoke class="VI" method="FP.Close"() -> ()  [unwired: 3 in, 3 out]
          }
          frame True {
          }
        }
      }
    }
  }
  n249 = while {
    tunnel: w1 -> [w604]
    stop <- w605 stop-if-true
    n250 = event shown="[2] \"Upload\": Value Change" {
      selector: _ -> [_ _ _ _ _ _ _ _ _]
      dyn-events: _ -> [_ _ _ _ _ _ _ _ _]
      timeout: _ -> [_ _ _ _ _ _ _ _ _]
      tunnel: [_ _ _ TRUE _ _ _ _ TRUE] -> w605
      tunnel: w604 -> [w607 _ w626 w632 _ w646 _ w648 w650]
      event "Flight Control Board": Value Change {
        n251 = event-data() -> ()  [unwired: 1 in, 1 out]
        n252 = Enqueue Element(queue=w607, element="Update Flight Options") -> ()  [unwired: 2 in, 3 out]
      }
      event "Next", "Previous": Value Change {
        n253 = event-data() -> ()  [unwired: 1 in, 1 out]
        n254 = local read "FlightConfig"() -> (w619:u16)
        n255 = property on="FlightConfig" class="Ring (strict)"() -> ("NumItems"=w617:u32)  [unwired: 2 in, 2 out]
        n256 = Increment(x=w619) -> (x+1=w621:u16)
        n257 = To Unsigned Word Integer(number=w617) -> (unsigned 16bit integer=w609:u16)
        n258 = Select(t=w621, s="Next", f=w619) -> (s? t:f=w614:u16)
        n259 = Equal?(x=w609, y=w614) -> (x = y?=w616:bool)
        n260 = Select(t=u16 0 ("unsigned 16bit integer"), s=w616, f=w614) -> (s? t:f=w613:u16)
        n261 = Decrement(x=w613) -> (x-1=w618:u16)
        n262 = Select(t=w618, s="Previous", f=w613) -> (s? t:f=w608:u16)
        n263 = Decrement(x=w609) -> (x-1=w611:u16)
        n264 = Greater?(x=w608, y=w609) -> (0:w610:bool)
        n265 = Select(t=w611, s=w610, f=w608) -> (s? t:f=w612:u16)
        n266 = local write "FlightConfig"(w612) -> ()
      }
      event "Upload": Value Change {
        n267 = event-data() -> ()  [unwired: 1 in, 1 out]
        n268 = local read "Com Port"() -> (w625:refnum<visa-resource-name>)
        n269 = Equal?(x=refnum<visa-resource-name> "<Select Com Port>" ("Com Port"), y=w625) -> (x = y?=w623:bool)
        n270 = case shown="False" w623 {
          tunnel: w626 -> [w628 _]
          frame False {
            n271 = Enqueue Element(queue=w628, element="Verify Serial Port") -> ()  [unwired: 2 in, 3 out]
          }
          frame True {
            n272 = One Button Dialog(message="Select COM port") -> ()  [unwired: 1 in, 1 out]
          }
        }
      }
      event Panel Close? {
        n273 = event-data() -> ()  [unwired: 1 in, 3 out]
        n274 = Enqueue Element(queue=w632, element="Exit") -> ()  [unwired: 2 in, 3 out]
        n275 = event-data("Discard?"=TRUE) -> ()  [unwired: 1 in, 1 out]
      }
      event "Options": Double Click; "Options": Mouse Down {
        n276 = event-data() -> ("Coords.Horizontal"=w636:i32)  [unwired: 1 in]
        n277 = Less Or Equal?(x=w636, y=25) -> (x <= y?=w634:bool)
        n278 = case shown="True" w634 {
          frame False {
          }
          frame True {
            w642 = 40
            n279 = property on="Options" class="LstBox (strict)"() -> ("Item Symbols"=w639:i32[], "Value"=w637:i32)  [unwired: 2 in, 2 out]
            n280 = Index Array(array=w639, index=w637) -> (element=w644:i32)
            n281 = Equal?(x=w644, y=w642) -> (x = y?=w643:bool)
            n282 = Select(t=39, s=w643, f=w642) -> (s? t:f=w640:i32)
            n283 = Replace Array Subset(array=w639, new element=w640, index=w637) -> (w638:i32[])
            n284 = property on="Options" class="LstBox (strict)"("Item Symbols"=w638) -> ()  [unwired: 2 in, 2 out]
          }
        }
      }
      event "Options": Value Change {
        n285 = event-data() -> ()  [unwired: 1 in, 1 out]
        n286 = Enqueue Element(queue=w646, element="Update Flight Option Description") -> ()  [unwired: 2 in, 3 out]
      }
      event "Update": Value Change {
        n287 = event-data() -> ()  [unwired: 1 in, 1 out]
        n288 = One Button Dialog(message="This will query the download server to check if a new version of the flight software is available.  This feature is currently under construction.") -> ()  [unwired: 1 in, 1 out]
      }
      event "Settings": Value Change {
        n289 = event-data() -> ()  [unwired: 1 in, 1 out]
        n290 = Enqueue Element(queue=w648, element="Update Settings") -> ()  [unwired: 2 in, 3 out]
      }
      event "Done": Value Change {
        n291 = event-data() -> ()  [unwired: 1 in, 1 out]
        n292 = Enqueue Element(queue=w650, element="Exit") -> ()  [unwired: 2 in, 3 out]
      }
    }
  }
